vi "[r]GET Decimal Array from Rows.vi"(7 "Filters":T1[](array[typedef]), 8 "Error in":errorcluster caption="Error in (no error)", 10 "$Path or Item Name":string="$[*].Contains[*].id", 11 "Table ID":u32=701) -> (0 "Error out":errorcluster, 3 "Requested Decimals Array":i32[](array[numeric])=[59, 228, 226, 220, 223, 231, 220])   [LabVIEW 2018]
uses:
  TypeDef/FIlter.ctl
  <vilib>/JDP Science/JSONtext/Next JSON Value.vi
  <vilib>/JDP Science/JSONtext/String Subset.vi
  <vilib>/JDP Science/JSONtext/support/Strip Quotes and Unescape.vi
  <vilib>/JDP Science/JSONtext/Parsing/Advance past next JSON Value (inlined COPY).vi
  <vilib>/JDP Science/JSONtext/support/Unescape JSON string.vi
  <vilib>/JDP Science/JSONtext/Parsing/Advance past whitespace.vi
  <vilib>/JDP Science/JSONtext/Parsing/Advance past String.vi
  <vilib>/JDP Science/JSONtext/Parsing/Advance past Number.vi
  <vilib>/JDP Science/JSONtext/Parsing/Advance past Line Ending.vi
  Collect Param - Bool.vi
  Collect Param - String.vi
  Collect Param - Decimal.vi
  <vilib>/JDP Science/JSONtext/Parsing/Parse Full Path or Item Name.vi
  <vilib>/JDP Science/JSONtext/Parsing/Advance past Array.vi
  <vilib>/JDP Science/JSONtext/Parsing/Advance past Object.vi
  <vilib>/JDP Science/JSONtext/support/Error Cluster From Code.vi
  <vilib>/JDP Science/JSONtext/Offset/Find Item Locations by Path.vi
  <vilib>/httpClient/LabVIEWHTTPClient.lvlib
  <vilib>/JDP Science/JSONtext/JSONtext.lvlib
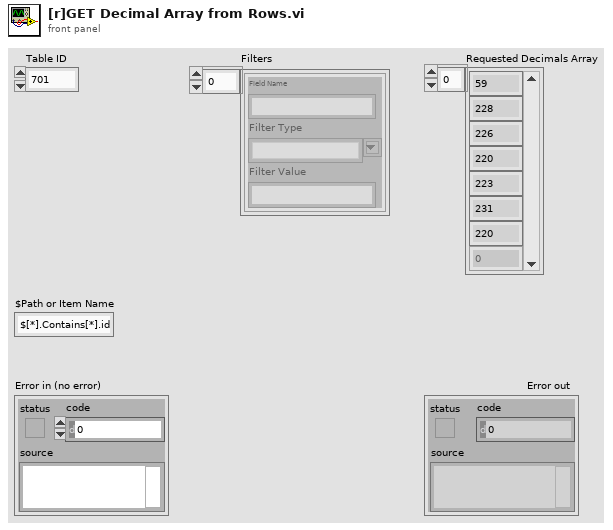
[diagram p1: front panel]
types:
  T1 = typedef "FIlter.ctl" = cluster{"Field Name":string, "Filter Type":string, "Filter Value":string}
  T2 = typedef "LabVIEWHTTPClient.lvlib/ClientHandle.ctl" = refnum<k1>
  T3 = typedef "Param.ctl" = cluster{"Param":string, "Value":string}
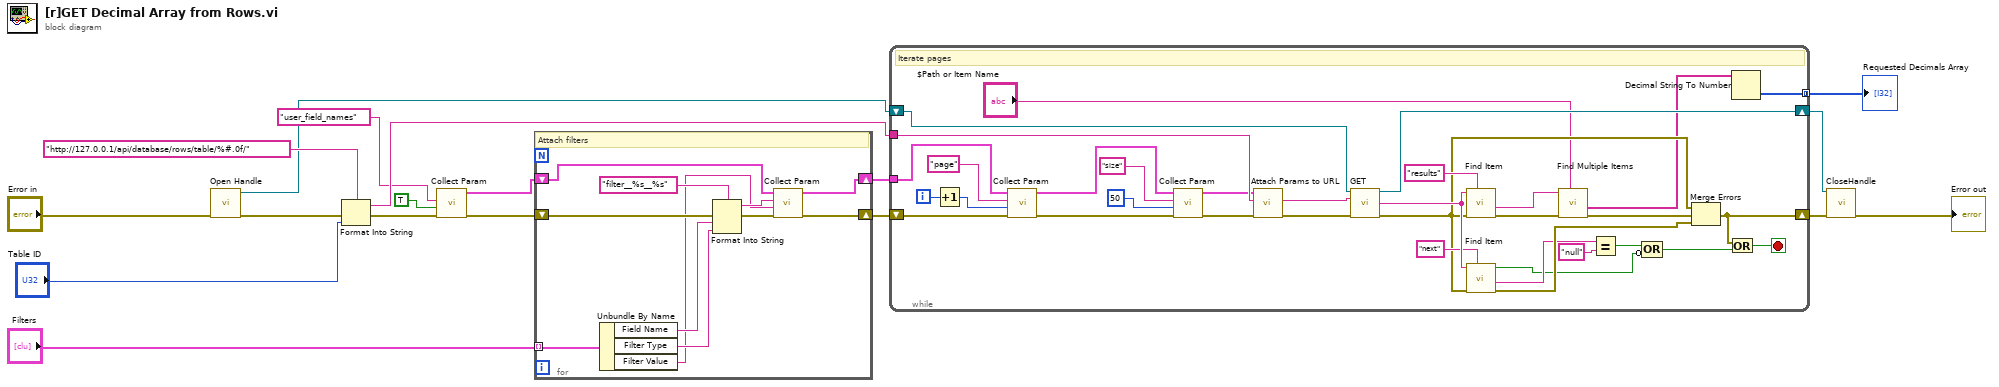
[diagram p0: block diagram]
diagram:
  n1 = call "Open Handle.vi"("error in (no error)"="Error in") -> ("error out"=w13:errorcluster, "Refnum out"=w12:T2)  [unwired: 9 in]
  n2 = Format Into String(format string="http://127.0.0.1/api/database/rows/table/%#.0f/" ("url"), error in=w13, "Table ID") -> (resulting string=w18:string, error out=w3:errorcluster)  [unwired: 1 in]
  n3 = call-poly "Collect Param.vi"("Error in"=w3, "Value"=TRUE, "Param Name"="user_field_names") -> ("Error out"=w2:errorcluster, "Params Array Out"=w5:T3[])  [unwired: 7 in]
  n4 = for {
    shift-right: [w28] -> w4
    shift-left: w5 -> [w29]
    shift-right: [w27] -> w1
    shift-left: w2 -> [w25]
    tunnel: "Filters" -> [w22] mode=indexing
    # "Attach filters"
    n5 = Unbundle By Name(w22) -> ("Field Name"=w21:string, "Filter Type"=w20:string, "Filter Value"=w19:string)
    n6 = Format Into String(format string="filter__%s__%s", error in=w25, w21, w20) -> (resulting string=w23:string, error out=w24:errorcluster)  [unwired: 1 in]
    n7 = call-poly "Collect Param.vi"("Error in"=w24, "Value"=w19, "Param Name"=w23, "Params Array In"=w29) -> ("Error out"=w27:errorcluster, "Params Array Out"=w28:T3[])  [unwired: 6 in]
  }
  n8 = while {
    tunnel: [w38] -> w9 mode=concatenating
    shift-right: [w62] -> w14
    shift-left: w12 -> [w63]
    shift-right: [w56] -> w15
    shift-left: w1 -> [w33]
    tunnel: w18 -> [w44]
    tunnel: w4 -> [w35]
    i -> [w42]
    stop <- w51 stop-if-true
    # "Iterate pages"
    n9 = Increment(x=w42) -> (x+1=w41:i32)
    n10 = call-poly "Collect Param.vi"("Error in"=w33, "Value"=w41, "Param Name"="page" ("Param"), "Params Array In"=w35) -> ("Error out"=w45:errorcluster, "Params Array Out"=w48:T3[])  [unwired: 6 in]
    n11 = call-poly "Collect Param.vi"("Error in"=w45, "Value"=50, "Param Name"="size" ("Param"), "Params Array In"=w48) -> ("Error out"=w32:errorcluster, "Params Array Out"=w34:T3[])  [unwired: 6 in]
    n12 = call "Attach Params to URL.vi"("Error in"=w32, "URL"=w44, "Param array"=w34) -> ("Error out"=w39:errorcluster, "URL with params"=w40:string)  [unwired: 7 in]
    n13 = call <vilib>:"GET.vi"("client handle"=w63, "url"=w40, "error in (no error)"=w39) -> ("client handle out"=w62:T2, "body"=w59:string, "error out"=w54:errorcluster)  [unwired: 9 in, 1 out]
    n14 = call <vilib>:"Find Item.vi"("$Path or Item Name"="results", "error in (no error)"=w54, "JSON"=w59) -> ("error out"=w57:errorcluster, "<JSON>"=w60:string)  [unwired: 5 in, 2 out]
    n15 = call <vilib>:"Find Item.vi"("$Path or Item Name"="next", "error in (no error)"=w54, "JSON"=w59) -> ("error out"=w53:errorcluster, "<JSON>"=w50:string, "Found"=w30:bool)  [unwired: 5 in, 1 out]
    n16 = call <vilib>:"Find Multiple Items.vi"("$Path or Item Name"="$Path or Item Name", "error in (no error)"=w57, "JSON"=w60) -> ("error out"=w55:errorcluster, "<JSON>"=w36:string[])  [unwired: 5 in, 2 out]
    n17 = Equal?(x=w50, y="null" ("x")) -> (x = y?=w52:bool)
    n18 = Compound Arithmetic op=OR(w52, invert w30) -> (w31:bool)
    n19 = Merge Errors(w54, w55, w53) -> (w56:errorcluster)
    n20 = Or(x=w56, y=w31) -> (x .or. y?=w51:bool)
    n21 = Decimal String To Number(string=w36) -> (number=w38:i32[])  [unwired: 2 in, 1 out]
  }
  "Requested Decimals Array" <- w9
  n22 = call <vilib>:"CloseHandle.vi"("client handle"=w14, "error in (no error)"=w15) -> ("error out"=→"Error out":errorcluster)  [unwired: 13 in]
